vi "Coverage Analyzer View.vi"(8 "error in (no error)":errorcluster, 11 "Coverage Analyzer Result View.lvclass":refnum<class "Coverage Analyzer Result View.lvclass">) -> (0 "error out":errorcluster)   [LabVIEW 2020, in "Coverage Analyzer.lvlib" / "Coverage Analyzer Result View.lvclass"]
uses:
  Coverage Analyzer Result View.lvclass
  Coverage Analyzer Result View.lvclass/Coverage Analyzer Result View.ctl
  fde09a69-7451-4da4-9368-3dcb0be6c936.vi
  <vilib>/Analysis/NI_AALBase.lvlib
  <vilib>/Analysis/baseanly.llb/Mean (DBL).vi
panel:
  in  "Method Test Times":i32(listbox)
  out "Debug disabled VIs":string
  out "Coverage for Executed VIs":string
  out "Fraction of VIs Executed":string
  in  "Hide VIs not executed?":bool=TRUE
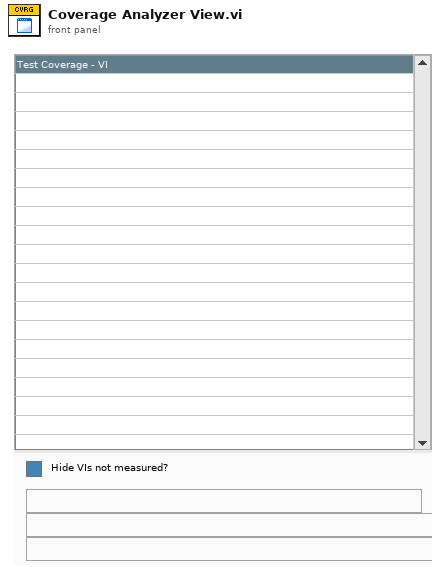
[diagram p1: front panel]
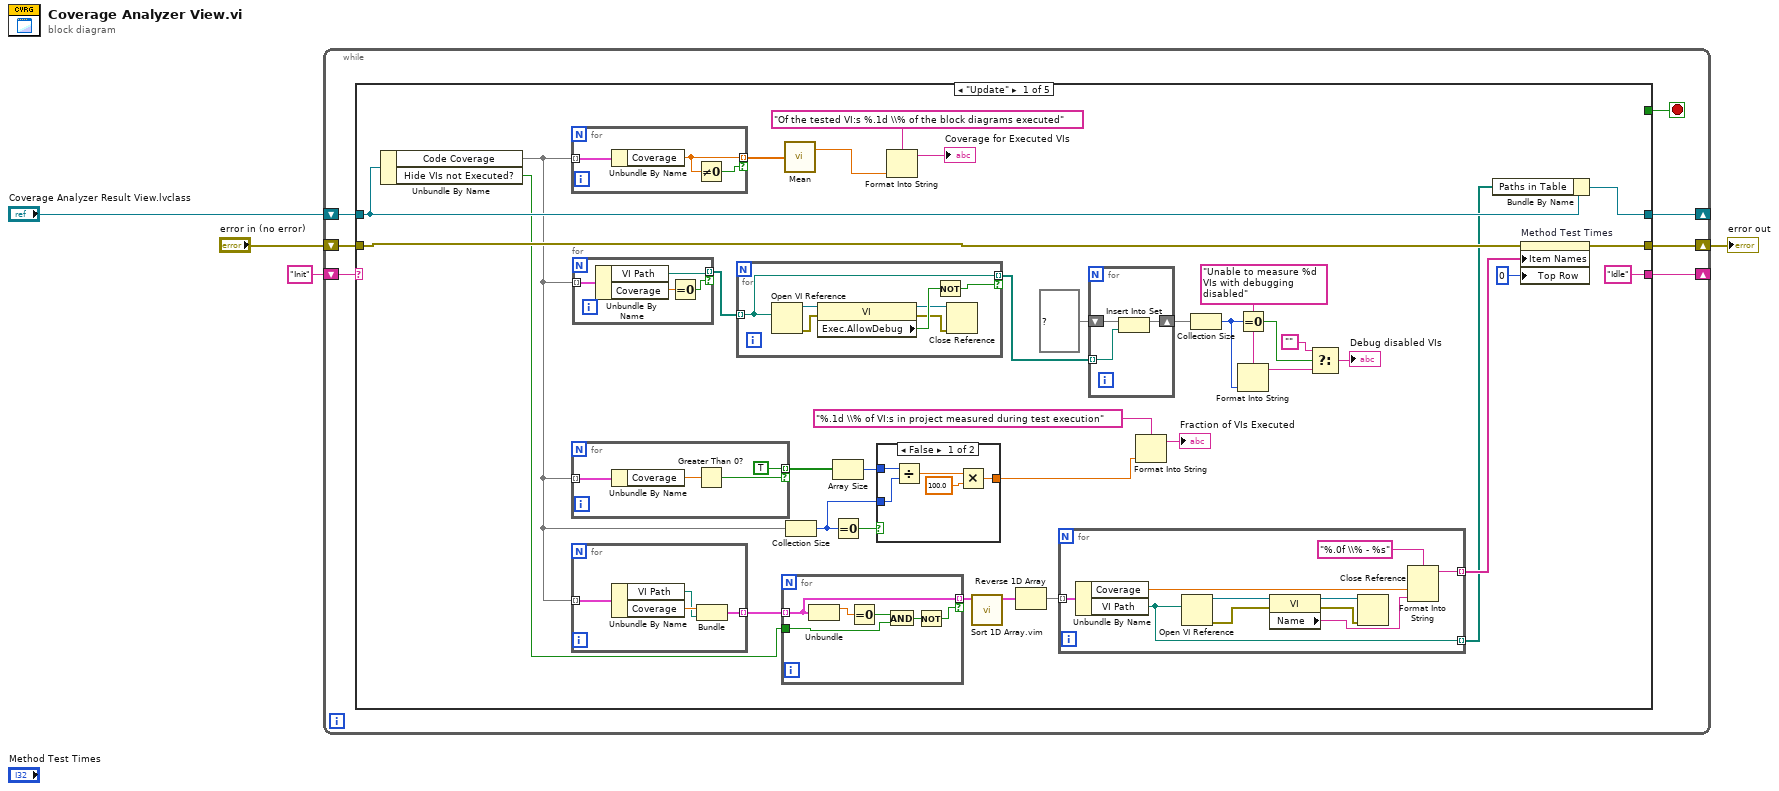
[diagram p0: block diagram]
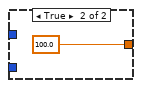
[diagram p2: hidden frame]
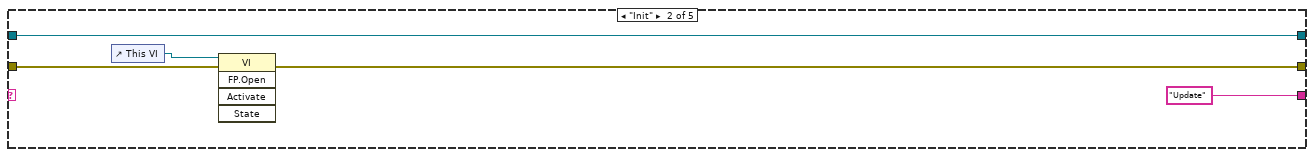
[diagram p3: hidden frame]
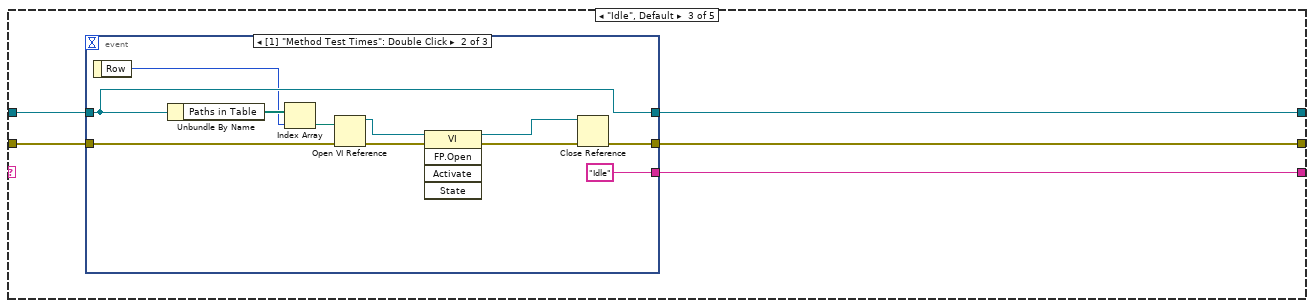
[diagram p4: hidden frame]
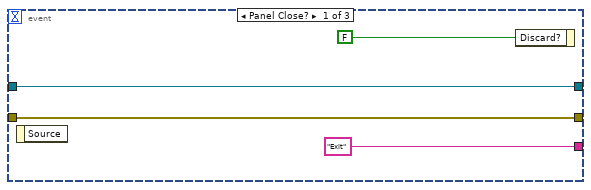
[diagram p5: hidden frame]
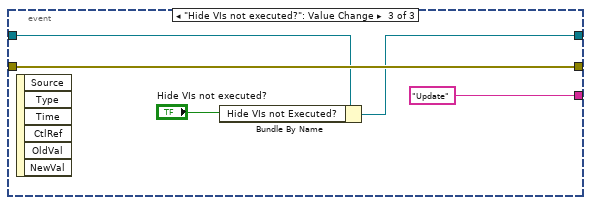
[diagram p6: hidden frame]
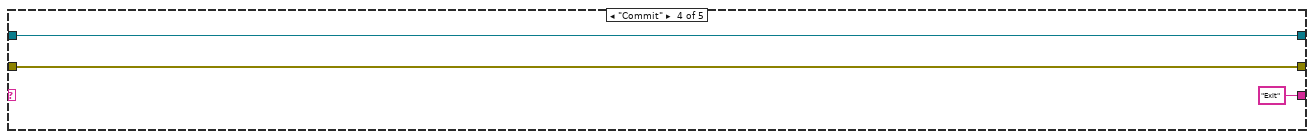
[diagram p7: hidden frame]
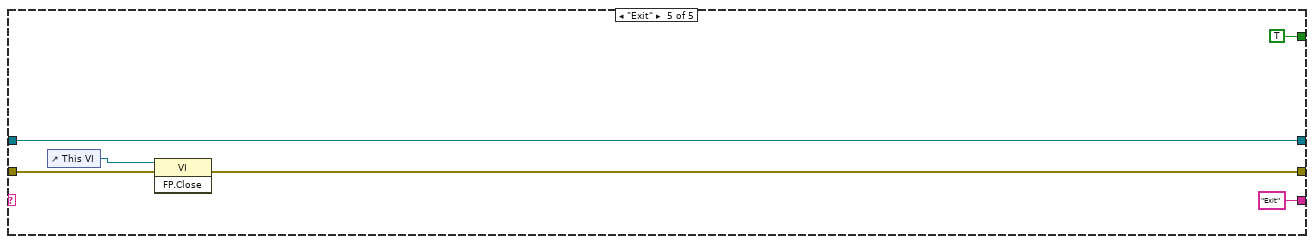
[diagram p8: hidden frame]
diagram:
  n1 = while {
    shift-right: [w8] -> _
    shift-left: "Coverage Analyzer Result View.lvclass" -> [w9]
    shift-right: [w5] -> w2
    shift-left: "error in (no error)" -> [w10]
    shift-right: [w7] -> _
    shift-left: "Init" -> [w11]
    stop <- w6 stop-if-true
    n2 = case shown="\"Update\"" w11 {
      tunnel: [w45 w96 w103 w126 w128] -> w5
      tunnel: w10 -> [w41 w95 w102 w126 w127]
      tunnel: w9 -> [w38 w94 w101 w125 w132]
      tunnel: [w43 w94 w100 w125 w132] -> w8
      tunnel: ["Idle" "Update" w99 "Exit" "Exit"] -> w7
      tunnel: [_ _ _ _ TRUE] -> w6
      frame "Update" {
        n3 = Unbundle By Name(w38) -> ("Code Coverage"=w13:map{path, dbl}, "Hide VIs not Executed?"=w12:bool)
        n4 = for {
          tunnel: w13 -> [w63] mode=indexing
          tunnel: [w62] -> w24 mode=indexing if=w61
          n5 = Unbundle By Name(w63) -> ("Coverage"=w62:dbl)
          n6 = Not Equal To 0?(x=w62) -> (x != 0?=w61:bool)
        }
        n7 = for {
          tunnel: w13 -> [w67] mode=indexing
          tunnel: [TRUE] -> w30 mode=indexing if=w64
          n8 = Unbundle By Name(w67) -> ("Coverage"=w66:dbl)
          n9 = Greater Than 0?(x=w66) -> (x > 0?=w64:bool)
        }
        n10 = for {
          tunnel: w13 -> [w83] mode=indexing
          tunnel: [w81] -> w35 mode=indexing
          n11 = Unbundle By Name(w83) -> ("VI Path"=w80:path, "Coverage"=w82:dbl)
          n12 = Bundle("Coverage"=w82, "VI Path"=w80) -> (w81:cluster{"Coverage":dbl, "VI Path":path})  [unwired: 1 in]
        }
        n13 = for {
          tunnel: w13 -> [w60] mode=indexing
          tunnel: [w57] -> w14 mode=indexing if=w58
          n14 = Unbundle By Name(w60) -> ("VI Path"=w57:path, "Coverage"=w59:dbl)
          n15 = Equal To 0?(x=w59) -> (x = 0?=w58:bool)
        }
        n16 = for {
          tunnel: w14 -> [w51] mode=indexing
          tunnel: [w51] -> w16 mode=indexing if=w50
          n17 = Open VI Reference(vi path=w51) -> (vi reference=w56:refnum<vi>, error out=w55:errorcluster)  [unwired: 5 in]
          n18 = property class="VI"(reference=w56, error in=w55) -> (reference out=w52:refnum<vi>, error out=w53:errorcluster, "Exec.AllowDebug"=w54:bool)
          n19 = Not(x=w54) -> (.not. x?=w50:bool)
          n20 = Close Reference(reference=w52, error in (no error)=w53) -> ()  [unwired: 1 out]
        }
        n21 = for {
          tunnel: [w79] -> w36 mode=indexing if=w74
          tunnel: w35 -> [w79] mode=indexing
          tunnel: w12 -> [w76]
          n22 = Unbundle(w79) -> ("Coverage"=w78:dbl)  [unwired: 1 out]
          n23 = Equal To 0?(x=w78) -> (x = 0?=w77:bool)
          n24 = And(x=w77, y=w76) -> (x .and. y?=w75:bool)
          n25 = Not(x=w75) -> (.not. x?=w74:bool)
        }
        n26 = call-poly <vilib>:"Mean.vi"("X"=w24) -> ("mean"=w25:dbl)  [unwired: 1 out]
        n27 = Collection Size(1:w13) -> (0:w28:i32)
        n28 = Array Size(array=w30) -> (size(s)=w31:i32)
        n29 = Equal To 0?(x=w28) -> (x = 0?=w27:bool)
        n30 = case shown="False" w27 {
          tunnel: w31 -> [w72 _]
          tunnel: [w69 100.0] -> w29
          tunnel: w28 -> [w70 _]
          frame False {
            n31 = Divide(x=w72, y=w70) -> (x/y=w71:dbl)
            n32 = Multiply(x=w71, y=100.0) -> (x*y=w69:dbl)
          }
          frame True {
          }
        }
        n33 = Format Into String(format string="Of the tested VI:s %.1d \\% of the block diagrams executed", w25) -> (resulting string=→"Coverage for Executed VIs":string)  [unwired: 2 in, 1 out]
        n34 = call "Sort 1D Array.vim"("unsorted array"=w36) -> ("sorted array"=w32:cluster{"Coverage":dbl, "VI Path":path}[])  [unwired: 10 in]
        n35 = Reverse 1D Array(array=w32) -> (reversed array=w33:cluster{"Coverage":dbl, "VI Path":path}[])
        n36 = for {
          tunnel: w33 -> [w93] mode=indexing
          tunnel: [w90] -> w44 mode=indexing
          tunnel: [w85] -> w34 mode=indexing
          n37 = Unbundle By Name(w93) -> ("Coverage"=w91:dbl, "VI Path"=w85:path)
          n38 = Open VI Reference(vi path=w85) -> (vi reference=w89:refnum<vi>, error out=w88:errorcluster)  [unwired: 5 in]
          n39 = property class="VI"(reference=w89, error in=w88) -> (reference out=w87:refnum<vi>, error out=w86:errorcluster, "Name"=w84:string)
          n40 = Close Reference(reference=w87, error in (no error)=w86) -> ()  [unwired: 1 out]
          n41 = Format Into String(format string="%.0f \\% - %s", w91, w84) -> (resulting string=w90:string)  [unwired: 2 in, 1 out]
        }
        n42 = for {
          shift-right: [w48] -> w18
          shift-left: set{path} {} ("VIs") -> [w49]
          tunnel: w16 -> [w47] mode=indexing
          n43 = Insert Into Set(10:w47, 11:w49) -> (3:w48:set{path})  [unwired: 1 out]
        }
        n44 = Format Into String(format string="%.1d \\% of VI:s in project measured during test execution", w29) -> (resulting string=→"Fraction of VIs Executed":string)  [unwired: 2 in, 1 out]
        n45 = Collection Size(1:w18) -> (0:w20:i32)
        n46 = Equal To 0?(x=w20) -> (x = 0?=w19:bool)
        n47 = Format Into String(format string="Unable to measure %d VIs with debugging disabled", w20) -> (resulting string=w21:string)  [unwired: 2 in, 1 out]
        n48 = Select(t="", s=w19, f=w21) -> (s? t:f=→"Debug disabled VIs":string)
        n49 = Bundle By Name(cluster=w38, "Paths in Table"=w34) -> (w43:refnum<class "Coverage Analyzer Result View.lvclass">)
        n50 = property on="Method Test Times" class="LstBox (strict)"(error in=w41, "Item Names"=w44, "Top Row"=0) -> (error out=w45:errorcluster)  [unwired: 1 in, 1 out]
      }
      frame "Init" {
        n51 = control-ref of="This VI"() -> (w97:refnum<vi>)
        n52 = invoke class="VI" method="FP.Open"(reference=w97, error in=w95) -> (error out=w96:errorcluster)  [unwired: 3 in, 4 out]
      }
      frame "Idle", Default {
        n53 = event shown="[1] \"Method Test Times\": Double Click" {
          selector: _ -> [_ _ _]
          dyn-events: _ -> [_ _ _]
          timeout: _ -> [_ _ _]
          tunnel: [w107 w109 w123] -> w103
          tunnel: w102 -> [w107 w108 w123]
          tunnel: w101 -> [w106 w117 w122]
          tunnel: [w106 w117 w120] -> w100
          tunnel: ["Exit" "Idle" "Update"] -> w99
          event Panel Close? {
            n54 = event-data() -> ()  [unwired: 1 in, 1 out]
            n55 = event-data("Discard?"=FALSE) -> ()  [unwired: 1 in, 1 out]
          }
          event "Method Test Times": Double Click {
            n56 = event-data() -> ("Row"=w115:i32)  [unwired: 1 in]
            n57 = Unbundle By Name(w117) -> ("Paths in Table"=w116:path[])
            n58 = Index Array(array=w116, index=w115) -> (element=w114:path)
            n59 = Open VI Reference(vi path=w114, error in (no error)=w108) -> (vi reference=w113:refnum<vi>, error out=w112:errorcluster)  [unwired: 4 in]
            n60 = invoke class="VI" method="FP.Open"(reference=w113, error in=w112) -> (reference out=w111:refnum<vi>, error out=w110:errorcluster)  [unwired: 3 in, 3 out]
            n61 = Close Reference(reference=w111, error in (no error)=w110) -> (error out=w109:errorcluster)
          }
          event "Hide VIs not executed?": Value Change {
            n62 = event-data() -> ()  [unwired: 1 in, 6 out]
            n63 = Bundle By Name(cluster=w122, "Hide VIs not Executed?"="Hide VIs not executed?") -> (w120:refnum<class "Coverage Analyzer Result View.lvclass">)
          }
        }
      }
      frame "Commit" {
      }
      frame "Exit" {
        n64 = control-ref of="This VI"() -> (w129:refnum<vi>)
        n65 = invoke class="VI" method="FP.Close"(reference=w129, error in=w127) -> (error out=w128:errorcluster)  [unwired: 1 in, 2 out]
      }
    }
  }
  "error out" <- w2
